vi "Accept Run.vi"(8 "error in (no error)":errorcluster, 9 "Ignore":bool, 10 "Accepted Runes":string, 11 "JSON Lexer in":refnum<class "JSON Lexer.lvclass">) -> (0 "error out":errorcluster, 3 "JSON Lexer out":refnum<class "JSON Lexer.lvclass">)   [LabVIEW 2013, in "JKI JSON Serialization.lvlib" / "JSON Lexer.lvclass"]
uses:
  JSON Lexer.lvclass
  JSON Lexer.lvclass/JSON Lexer.ctl
  <vilib>/addons/_JKI.lib/Unicode/UTF-8 String/UTF-8 String.lvclass/UTF-8 String.ctl
  <vilib>/addons/_JKI.lib/Unicode/UTF-8 String/Index Rune as UTF-8 Substring.vi
  <vilib>/addons/_JKI.lib/Unicode/UTF-8 String/Next Rune As UTF-8 Substring.vi
  <vilib>/addons/_JKI.lib/Unicode/UTF-8 String/Bytes In Rune.vi
  <vilib>/Utility/error.llb/Error Cluster From Error Code.vi
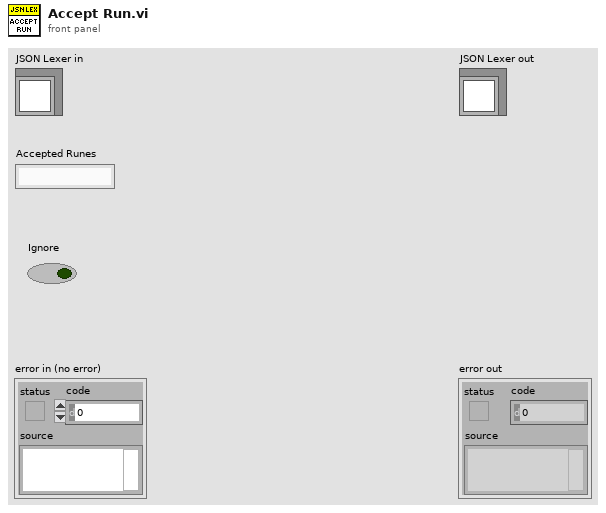
[diagram p1: front panel]
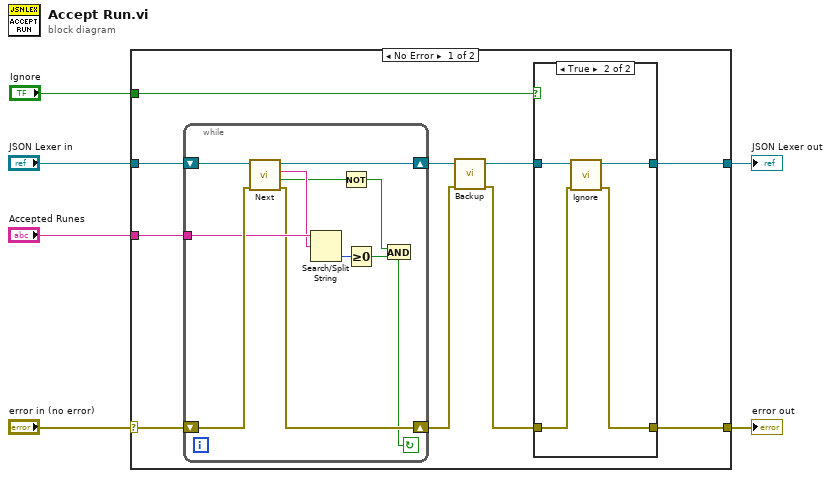
[diagram p0: block diagram]
diagram:
  n1 = case shown="No Error" "error in (no error)" {
    selector: "error in (no error)" -> [w15 w35]
    tunnel: [w8 w35] -> w5
    tunnel: [w10 w34] -> w3
    tunnel: "JSON Lexer in" -> [w16 w34]
    tunnel: "Accepted Runes" -> [w14 _]
    tunnel: "Ignore" -> [w7 _]
    frame No Error {
      n2 = while {
        tunnel: w14 -> [w31]
        shift-right: [w28] -> w12
        shift-left: w16 -> [w33]
        shift-right: [w29] -> w13
        shift-left: w15 -> [w32]
        stop <- w24 continue-if-true
        n3 = call "Next.vi"("error in (no error)"=w32, "JSON Lexer in"=w33) -> ("error out"=w29:errorcluster, "EOF"=w23:bool, "Rune"=w27:string, "JSON Lexer out"=w28:refnum<class "JSON Lexer.lvclass">)  [unwired: 6 in]
        n4 = Search/Split String(string=w31, search string/char (-)=w27) -> (offset of match=w30:i32)  [unwired: 1 in, 2 out]
        n5 = Not(x=w23) -> (.not. x?=w25:bool)
        n6 = Greater Or Equal To 0?(x=w30) -> (x >= 0?=w26:bool)
        n7 = And(x=w25, y=w26) -> (x .and. y?=w24:bool)
      }
      n8 = call "Backup.vi"("error in (no error)"=w13, "JSON Lexer in"=w12) -> ("error out"=w9:errorcluster, "JSON Lexer out"=w11:refnum<class "JSON Lexer.lvclass">)  [unwired: 8 in]
      n9 = case shown="True" w7 {
        tunnel: w11 -> [w18 w22]
        tunnel: [w18 w21] -> w10
        tunnel: w9 -> [w17 w20]
        tunnel: [w17 w19] -> w8
        frame False {
        }
        frame True {
          n10 = call "Ignore.vi"("error in (no error)"=w20, "JSON Lexer in"=w22) -> ("error out"=w19:errorcluster, "JSON Lexer out"=w21:refnum<class "JSON Lexer.lvclass">)  [unwired: 8 in]
        }
      }
    }
    frame Error {
    }
  }
  "error out" <- w5
  "JSON Lexer out" <- w3
